vi "PreInstall.vi"() -> (0 "error out":errorcluster)   [LabVIEW 2014]
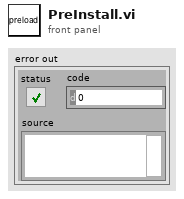
[diagram p1: front panel]
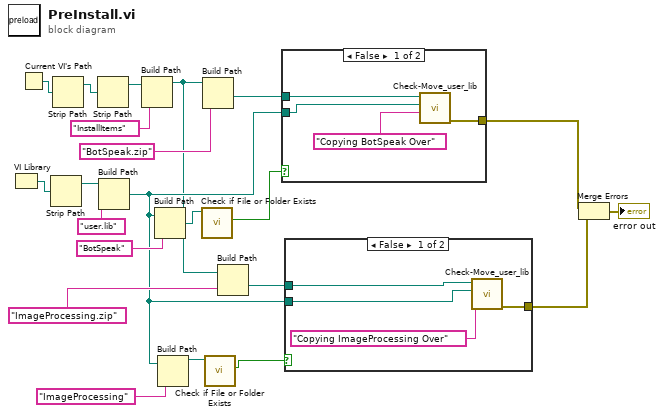
[diagram p0: block diagram]
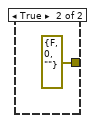
[diagram p2: hidden frame]
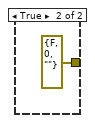
[diagram p3: hidden frame]
diagram:
  n1 = VI Library() -> (path=w17:path)
  n2 = Current VI's Path() -> (path=w13:path)
  n3 = Strip Path(path=w17) -> (stripped path=w19:path)  [unwired: 1 out]
  n4 = Strip Path(path=w13) -> (stripped path=w14:path)  [unwired: 1 out]
  n5 = Strip Path(path=w14) -> (stripped path=w6:path)  [unwired: 1 out]
  n6 = Build Path(base path=w19, name or relative path="user.lib") -> (appended path=w7:path)
  n7 = Build Path(base path=w6, name or relative path="InstallItems") -> (appended path=w5:path)
  n8 = Build Path(base path=w7, name or relative path="BotSpeak") -> (appended path=w21:path)
  n9 = Build Path(base path=w7, name or relative path="ImageProcessing") -> (appended path=w11:path)
  n10 = call <vilib>:"Check if File or Folder Exists.vi"("path"=w21) -> ("file or folder exists?"=w22:bool)  [unwired: 8 in, 2 out]
  n11 = Build Path(base path=w5, name or relative path="BotSpeak.zip") -> (appended path=w16:path)
  n12 = call <vilib>:"Check if File or Folder Exists.vi"("path"=w11) -> ("file or folder exists?"=w10:bool)  [unwired: 8 in, 2 out]
  n13 = Build Path(base path=w5, name or relative path="ImageProcessing.zip") -> (appended path=w8:path)
  n14 = case shown="False" w22 {
    tunnel: w16 -> [w26 _]
    tunnel: w7 -> [w25 _]
    tunnel: [w23 errorcluster {"status"=FALSE, "code"=0, "source"=""} ("error out")] -> w3
    frame False {
      n15 = call "Check-Move_user_lib.vi"("message"="Copying BotSpeak Over", "Target"=w25, "ZIP FILE"=w26) -> ("error out"=w23:errorcluster)  [unwired: 8 in]
    }
    frame True {
    }
  }
  n16 = case shown="False" w10 {
    tunnel: w8 -> [w31 _]
    tunnel: w7 -> [w30 _]
    tunnel: [w28 errorcluster {"status"=FALSE, "code"=0, "source"=""} ("error out")] -> w2
    frame False {
      n17 = call "Check-Move_user_lib.vi"("message"="Copying ImageProcessing Over", "Target"=w30, "ZIP FILE"=w31) -> ("error out"=w28:errorcluster)  [unwired: 8 in]
    }
    frame True {
    }
  }
  n18 = Merge Errors(w3, w2) -> (→"error out":errorcluster)
